vi "Example.vi"(3 "stop":bool) -> (1 "error out":errorcluster)   [LabVIEW 2022 SP3, in "Logger.lvlib"]
uses:
  Logger.lvlib
  Logger/_Level.ctl
  FileHandler/FileHandler.lvclass
  C:/Users/jakub/repos/gh/sw4sys/lv-logger/Logger/Source/Handler/Handler.lvclass
  Logger/Logger.lvclass
  DateTime/Source/DateTime.lvlib
  Handler/Handler.lvclass
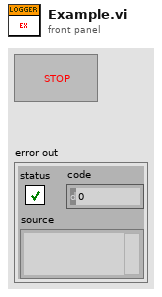
[diagram p1: front panel]
types:
  T1 = typedef "Logger.lvlib/Logger.lvclass/_Level.ctl" = enum16{"NOTSET", "DEBUG", "INFO", "WARNING", "ERROR", "CRITICAL"}
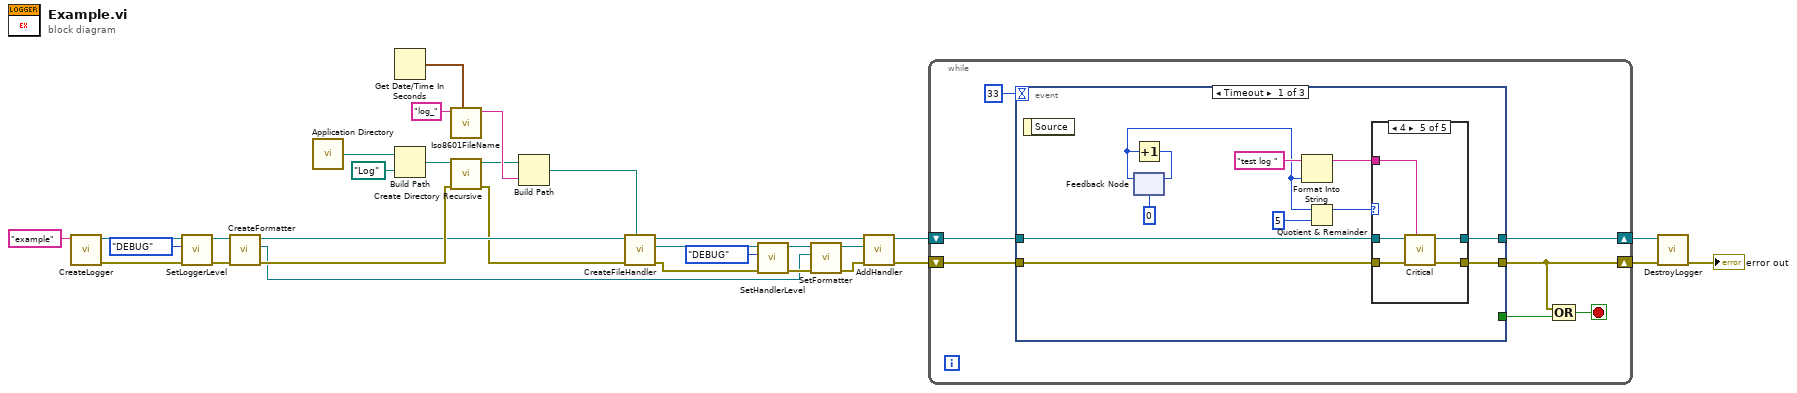
[diagram p0: block diagram]
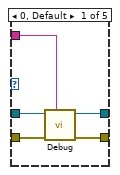
[diagram p2: hidden frame]
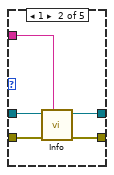
[diagram p3: hidden frame]
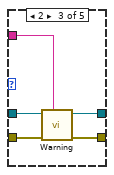
[diagram p4: hidden frame]
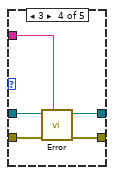
[diagram p5: hidden frame]
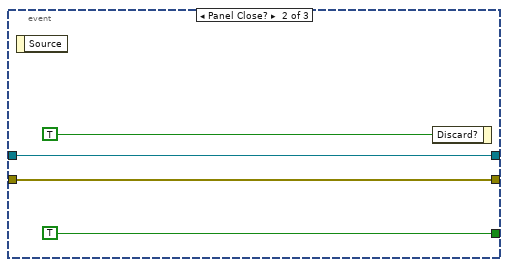
[diagram p6: hidden frame]
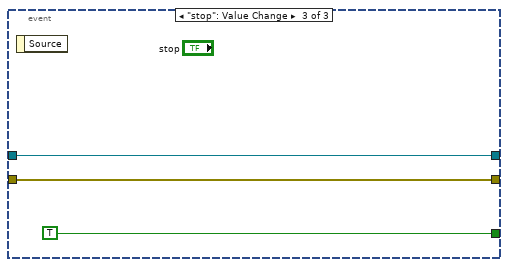
[diagram p7: hidden frame]
diagram:
  n1 = call "CreateLogger.vi"("Name"="example") -> ("error out"=w31:errorcluster, "Logger"=w23:refnum<class "Logger.lvclass">)  [unwired: 9 in]
  n2 = call-dynamic "SetLoggerLevel.vi"("error in (no error)"=w31, "Level"=_Level."DEBUG", "Logger in"=w23) -> ("error out"=w24:errorcluster, "Logger out"=w19:refnum<class "Logger.lvclass">)  [unwired: 7 in]
  n3 = call-dynamic "CreateFormatter.vi"("error in (no error)"=w24, "Logger in"=w19) -> ("error out"=w16:errorcluster, "Formatter"=w3:refnum<class "Formatter.lvclass">, "Logger out"=w11:refnum<class "Logger.lvclass">)  [unwired: 7 in]
  n4 = call <vilib>:"Application Directory.vi"() -> ("Application Directory"=w28:path)
  n5 = Get Date/Time In Seconds() -> (seconds since 1Jan1904=w5:timestamp)
  n6 = Build Path(base path=w28, name or relative path=path "Log") -> (appended path=w14:path)
  n7 = call "Iso8601FileName.vi"("TimeStamp"=w5, "Prefix ('')"="log_") -> ("FileName"=w13:string)  [unwired: 9 in]
  n8 = call <vilib>:"Create Directory Recursive.vi"("error in (no error)"=w16, "directory"=w14) -> ("error out"=w10:errorcluster, "directory copy"=w4:path)  [unwired: 3 in, 1 out]
  n9 = Build Path(base path=w4, name or relative path=w13) -> (appended path=w12:path)
  n10 = call-dynamic "CreateFileHandler.vi"("FIlePath"=w12, "error in (no error)"=w10, "Logger in"=w11) -> ("error out"=w29:errorcluster, "FileHandler"=w9:refnum<class "FileHandler.lvclass">, "Logger out"=w7:refnum<class "Logger.lvclass">)  [unwired: 6 in]
  n11 = call "SetHandlerLevel.vi"("error in (no error)"=w29, "Level"=_Level."DEBUG", "Handler in"=w9) -> ("error out"=w25:errorcluster, "Handler out"=w8:refnum<class "Handler.lvclass">)  [unwired: 7 in]
  n12 = call "SetFormatter.vi"("error in (no error)"=w25, "Formatter in"=w3, "Handler in"=w8) -> ("error out"=w18:errorcluster, "Handler out"=w17:refnum<class "Handler.lvclass">)  [unwired: 6 in, 1 out]
  n13 = call-dynamic "AddHandler.vi"("error in (no error)"=w18, "Handler in"=w17, "Logger in"=w7) -> ("error out"=w21:errorcluster, "Logger out"=w20:refnum<class "Logger.lvclass">)  [unwired: 6 in, 1 out]
  n14 = while {
    shift-right: [w36] -> w26
    shift-left: w20 -> [w38]
    shift-right: [w32] -> w27
    shift-left: w21 -> [w37]
    stop <- w34 stop-if-true
    n15 = event shown="[0] Timeout" {
      selector: _ -> [_ _ _]
      dyn-events: _ -> [_ _ _]
      timeout: 33 ("millisecond multiple") -> [_ _ _]
      tunnel: w38 -> [w49 w77 w81]
      tunnel: w37 -> [w48 w76 w80]
      tunnel: [w47 w77 w81] -> w36
      tunnel: [_ TRUE ("stop") TRUE ("stop")] -> w35
      tunnel: [w45 w76 w80] -> w32
      event Timeout {
        n16 = event-data() -> ()  [unwired: 1 in, 1 out]
        n17 = feedback #1(u32 0) -> (w39:u32)
        n18 = Increment(x=w39) -> (x+1=w40:u32)
        n19 = feedback-in #1(w40) -> ()
        n20 = Format Into String(initial string="test log ", w39) -> (resulting string=w42:string)  [unwired: 2 in, 1 out]
        n21 = Quotient & Remainder(x=w39, y=u32 5) -> (x-y*floor(x/y)=w43:u32)  [unwired: 1 out]
        n22 = case shown="4" w43 {
          tunnel: w49 -> [w52 w59 w62 w67 w72]
          tunnel: w48 -> [w54 w58 w64 w69 w74]
          tunnel: [w51 w57 w61 w66 w71] -> w47
          tunnel: [w53 w56 w63 w68 w73] -> w45
          tunnel: w42 -> [w50 w55 w60 w65 w70]
          frame 0, Default {
            n23 = call-dynamic "Debug.vi"("Message"=w50, "error in (no error)"=w54, "Logger in"=w52) -> ("error out"=w53:errorcluster, "Logger out"=w51:refnum<class "Logger.lvclass">)  [unwired: 7 in]
          }
          frame 1 {
            n24 = call-dynamic "Info.vi"("Message"=w55, "error in (no error)"=w58, "Logger in"=w59) -> ("error out"=w56:errorcluster, "Logger out"=w57:refnum<class "Logger.lvclass">)  [unwired: 7 in]
          }
          frame 2 {
            n25 = call-dynamic "Warning.vi"("Message"=w60, "error in (no error)"=w64, "Logger in"=w62) -> ("error out"=w63:errorcluster, "Logger out"=w61:refnum<class "Logger.lvclass">)  [unwired: 7 in]
          }
          frame 3 {
            n26 = call-dynamic "Error.vi"("Message"=w65, "error in (no error)"=w69, "Logger in"=w67) -> ("error out"=w68:errorcluster, "Logger out"=w66:refnum<class "Logger.lvclass">)  [unwired: 7 in]
          }
          frame 4 {
            n27 = call-dynamic "Critical.vi"("Message"=w70, "error in (no error)"=w74, "Logger in"=w72) -> ("error out"=w73:errorcluster, "Logger out"=w71:refnum<class "Logger.lvclass">)  [unwired: 7 in]
          }
        }
      }
      event Panel Close? {
        n28 = event-data() -> ()  [unwired: 1 in, 1 out]
        n29 = event-data("Discard?"=TRUE) -> ()  [unwired: 1 in, 1 out]
      }
      event "stop": Value Change {
        n30 = event-data() -> ()  [unwired: 1 in, 1 out]
      }
    }
    n31 = Compound Arithmetic op=OR(w32, w35) -> (w34:bool)
  }
  n32 = call-dynamic "DestroyLogger.vi"("error in (no error)"=w27, "Logger in"=w26) -> ("error out"=→"error out":errorcluster)  [unwired: 9 in]
